vi "MHX Overall Heat Transfer Coefficient.vi"(4 "MHX Tube Wall Thickness":dbl, 5 "MHX Tube h":dbl, 6 "MHX Shell h":dbl, 7 "Am":dbl, 9 "Thermal Conductivity of Hastealloy N":dbl, 10 "Ao":dbl, 11 "Ai":dbl) -> (3 "MHX Overall Heat Transfer Coefficient":dbl)   [LabVIEW 2019]
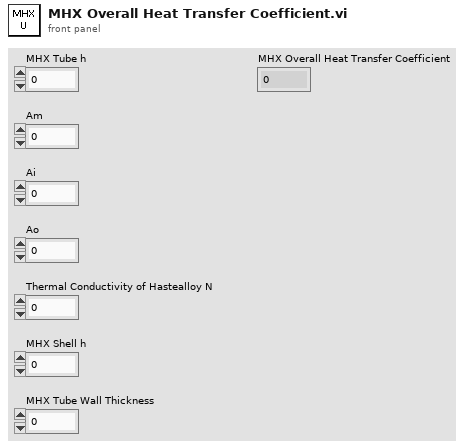
[diagram p1: front panel]
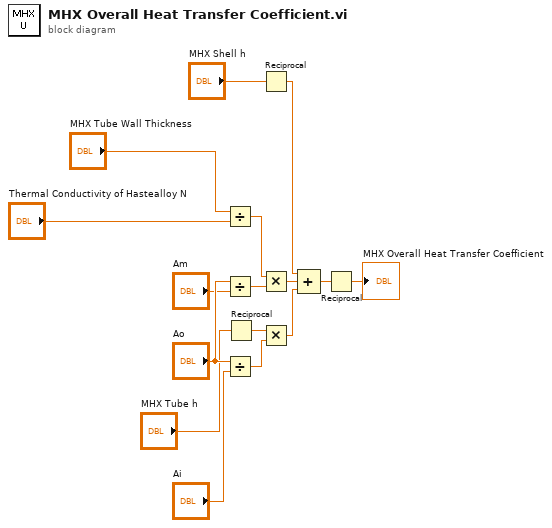
[diagram p0: block diagram]
diagram:
  n1 = Divide(x="MHX Tube Wall Thickness", y="Thermal Conductivity of Hastealloy N") -> (x/y=w5:dbl)
  n2 = Divide(x="Ao", y="Am") -> (x/y=w6:dbl)
  n3 = Divide(x="Ao", y="Ai") -> (x/y=w13:dbl)
  n4 = Reciprocal(x="MHX Tube h") -> (1/x=w12:dbl)
  n5 = Reciprocal(x="MHX Shell h") -> (1/x=w2:dbl)
  n6 = Multiply(x=w5, y=w6) -> (x*y=w7:dbl)
  n7 = Multiply(x=w12, y=w13) -> (x*y=w10:dbl)
  n8 = Compound Arithmetic op=ADD(w2, w7, w10) -> (w11:dbl)
  n9 = Reciprocal(x=w11) -> (1/x=→"MHX Overall Heat Transfer Coefficient":dbl)
